vi "Diagnostics.Protocol.Initialize.vi"(8 "error in (no error)":errorcluster, 11 "Parameters":T6={"Properties"={"Name"="", "CAN"={"Interface"="", "Baud Rate"=0, "Diagnostic Protocol"=enum."GMLAN", "Transport Protocol"=enum."ISO TP - Normal Mode", "Transmit ID"=0, "Receive ID"=0, "Transmit Extension"=0, "Receive Extension"=0, "Receive UUDT ID"=0, "Enable Stream"=FALSE, "VW TP Channel ID"=0, "Fill Frame"=FALSE, "Fill Byte"=0, "Termination"=FALSE, "LIN Cluster"="ADCS_LIN_database", "NAD"=1, "IO Mode"=0, "Max DLC"=8, "FD Baud Rate"=0, "Security"={"Type"=enum."None", "Source DLL Path"=path "", "Target DLL Path"=path "", "Security Level"=0, "Master Key"=""}, "Timeout"=0}, "986x"={"Enable"=FALSE, "RIO Device"="", "Bitfile"=path ""}, "Reads"=[], "Frames Lookup"=variant, "Writes"=[], "DPIDs"=[], "DPID Lookup"=variant, "DTC"={"Descriptor"={"DTC Byte Length"=0, "Status Byte Length"=0, "Add Data Byte Length"=0, "Byte Order"=enum."Motorola"}, "Value.Code"=[], "Value.String"=[], "Value.J2012String"=[], "Status.Code"=[], "Status.String"=[]}, "Created DTCs"=0, "Polls"=[], "Service Channels Status Lookup"=variant, "Trigger Lookup"=variant}} {"Properties"."Writes"."Signals"."Byte Order" items=["Little Endian", "Big Endian"]; "Properties"."Writes"."Signals"."Data Type" items=["Signed", "Unsigned", "IEEE Float"]; "Properties"."CAN"."IO Mode" items=["CAN 2.0", "CAN FD", "CAN FD+BRS"]; "Properties"."CAN"."Fill Byte" format="%.0x"; "Properties"."CAN"."VW TP Channel ID" format="%.0x"; "Properties"."CAN"."Receive UUDT ID" format="%.0x"; "Properties"."CAN"."Receive Extension" format="%.0x"; "Properties"."CAN"."Transmit Extension" format="%.0x"; "Properties"."CAN"."Receive ID" format="%.0x"; "Properties"."CAN"."Transmit ID" format="%.0x"; "Properties"."Reads"."Signals"."Byte Order" items=["Little Endian", "Big Endian"]; "Properties"."Reads"."Signals"."Data Type" items=["Signed", "Unsigned", "IEEE Float"]}) -> (0 "error out":errorcluster, 3 "diag ref out":T1={"Diag CAN Handle"=0, "Transport Protocol"=enum."ISO TP - Normal Mode", "Receive Address Extension"=0, "Transmit Address Extension"=0, "Receive CAN Id"=0, "Transmit CAN Id"=0, "Log Frames ?"=FALSE, "My TP Address"=0, "Other TP Address"=0, "T1"=0, "T2"=0, "T3"=0, "T4"=0, "Tx SN"=0, "Block Size"=0, "Rx SN"=0, "VW TP Initialized?"=FALSE, "Tx block no"=0, "baud rate"=0, "Interface"="", "Channel Diag CAN Handle"=0, "UDP Connection ID"=refnum, "TCP Connection ID"=refnum, "Target IP Addr"=0, "Source Address"=0, "Target Address"=0, "Send Header NACK?"=FALSE, "DLL Handle"=0, "NAD"=0, "Time Stamp read first"=0.0, "Time Stamp read last"=0.0, "Time Stamp write first"=0.0, "Time Stamp write last"=0.0, "Time Stamp write"=0.0, "Time Stamp read"=0.0, " I/O Mode"=0, "FD Baudrate"=0, "TX_DL"=8, "RX_DL"=8, "DoIP Protocol Version"=1, " Selected I/O Mode"=0, "TesterPresent Counter"=0, "TesterPresent Limit"=0, "TesterPresent Tick[ms]"=10, "TesterPresent RequireResponse?"=FALSE, "TesterPresent Stored Ref?"=FALSE, "TesterPresent Message"=[], "TesterPresent Task Handle"=0, "TesterPresent Semaphore"=refnum, "Response Plausibility Check"=1, "Default Version?"=TRUE, "Diagostic Globals"={"Timeout FC (Bs)"=250, "Timeout CF (Cr)"=250, "Timeout Diag Command"=1000, "Receive Block Size (BS)"=0, "Wait Time CF (STmin)"=5, "Max Waits (N_WFTmax)"=10, "Waits to Send (N_WAIT)"=0, "Time between Waits (TW)"=25, "Fill CAN Frames?"=TRUE, "Fill Byte"=255, "Invalid Response as Error?"=FALSE, "Max RspPending Count"=5, "VWTP Command Timeout"=50, "Transport Protocol"=enum."Diagnostics on IP", "Diag CAN Handle"=0, "DLL Handle"=0, "Timeout RspPending"=1000}, "Session-based Properties?"=FALSE} {"Diagostic Globals"."Fill Byte" format="%x"; "TesterPresent Message" format="%.0x"; "Selected I/O Mode" items=["CAN", "CAN FD", "CAN FD+BRS", "ECU Determined"]; "DoIP Protocol Version" items=["2010"=1, "2012"=2]; "RX_DL" items=["8"=8, "12"=12, "16"=16, "20"=20, "24"=24, "32"=32, "48"=48, "64"=64]; "TX_DL" items=["8"=8, "12"=12, "16"=16, "20"=20, "24"=24, "32"=32, "48"=48, "64"=64]; "I/O Mode" items=["CAN", "CAN FD", "CAN FD+BRS", "Not yet determined"]})   [LabVIEW 2019, in "Diagnostics Addon Engine.lvlib"]
uses:
  Diagnostics Addon Engine.lvlib
  Shared/Types/SysDef.Compile.ctl
  Shared/Types/SysDef.Compile.Properties.ctl
  Shared/Types/CAN.ctl
  Shared/Types/CAN.Interface.ctl
  Shared/Types/Protocol.ctl
  Shared/Types/Transport.ctl
  Shared/Types/Security.ctl
  Shared/Types/Security.Type.ctl
  Shared/Types/986x.ctl
  Shared/Types/Frame.Compile.ctl
  Shared/Types/Type.ctl
  Shared/Types/Signal.ctl
  Shared/Types/DPID.ctl
  Shared/Types/DPID.Rate.ctl
  Shared/Types/DTC.Settings.ctl
  Shared/Types/DTC.Descriptor.ctl
  Shared/Types/Poll.Compiled.ctl
  <vilib>/Automotive Diagnostic Command Set/Diagnostic Transport.llb/Diag Reference.ctl
  <vilib>/Automotive Diagnostic Command Set/Diagnostic Transport.llb/Transport Protocol Selector.ctl
  <vilib>/Automotive Diagnostic Command Set/Diagnostic Transport.llb/DoIP Protocol Version.ctl
  <vilib>/Automotive Diagnostic Command Set/Diagnostic Transport.llb/Diag Globals.ctl
  <vilib>/Automotive Diagnostic Command Set/Diagnostic Transport.llb/Property ID.ctl
  <vilib>/Automotive Diagnostic Command Set/Diagnostic Transport.llb/VWTP Application Type.ctl
  <vilib>/Automotive Diagnostic Command Set/Diagnostic Transport.llb/DoIP OpenType.ctl
  <vilib>/addons/Automotive Diagnostic Command Set/NI_Automotive Diagnostic Command Set.lvlib
  Shared/Diagnostics Addon Shared.lvlib
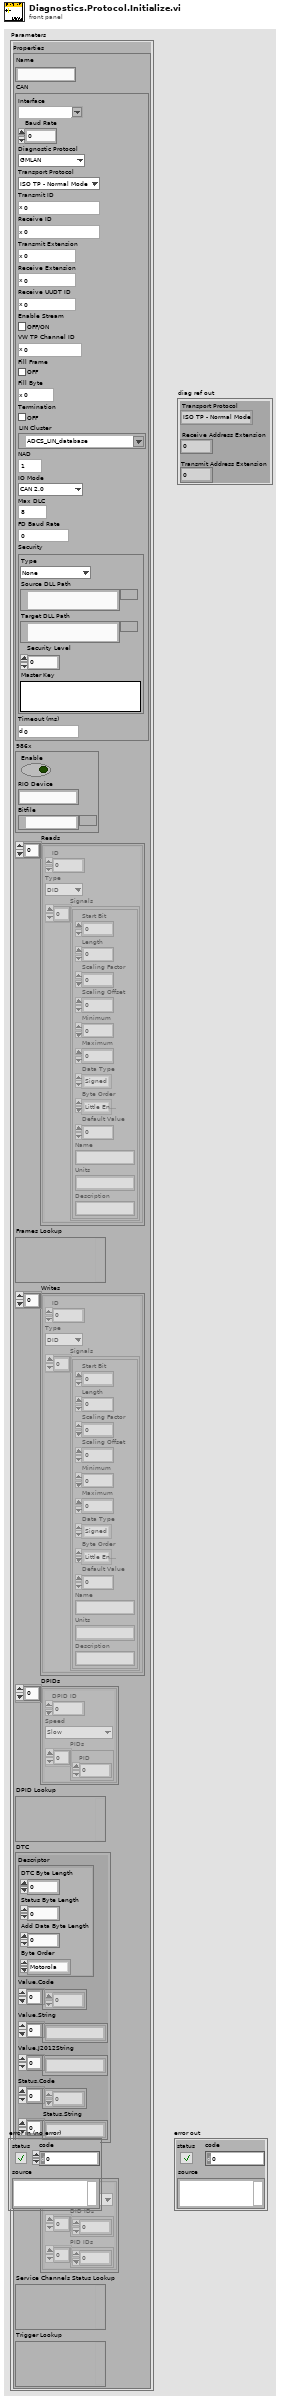
[diagram p1: front panel]
types:
  T1 = typedef "NI_Automotive Diagnostic Command Set.lvlib/Diag Reference.ctl" = cluster{"Diag CAN Handle":u32, "Transport Protocol":T2, "Receive Address Extension":u8, "Transmit Address Extension":u8, "Receive CAN Id":u32, "Transmit CAN Id":u32, "Log Frames ?":bool, "My TP Address":u8, "Other TP Address":u8, "T1":u16, "T2":u16, "T3":u16, "T4":u16, "Tx SN":u8, "Block Size":u8, "Rx SN":u8, "VW TP Initialized?":bool, "Tx block no":u8, "baud rate":u64, "Interface":string, "Channel Diag CAN Handle":u32, "UDP Connection ID":refnum<k16>, "TCP Connection ID":refnum<k5>, "Target IP Addr":u32, "Source Address":u16, "Target Address":u16, "Send Header NACK?":bool, "DLL Handle":u32, "NAD":u8, "Time Stamp read first":dbl, "Time Stamp read last":dbl, "Time Stamp write first":dbl, "Time Stamp write last":dbl, "Time Stamp write":dbl, "Time Stamp read":dbl, " I/O Mode":u32, "FD Baudrate":u64, "TX_DL":u16, "RX_DL":u16, "DoIP Protocol Version":T3, " Selected I/O Mode":u32, "TesterPresent Counter":u32, "TesterPresent Limit":u32, "TesterPresent Tick[ms]":i32, "TesterPresent RequireResponse?":bool, "TesterPresent Stored Ref?":bool, "TesterPresent Message":u8[], "TesterPresent Task Handle":i32, "TesterPresent Semaphore":T4, "Response Plausibility Check":u32, "Default Version?":bool, "Diagostic Globals":T5, "Session-based Properties?":bool}
  T2 = typedef "NI_Automotive Diagnostic Command Set.lvlib/Transport Protocol Selector.ctl" = enum16{"ISO TP - Normal Mode", "ISO TP - Mixed Mode", "VW TP 2.0", "Diagnostics on IP", "ISO TP LIN"}
  T3 = typedef "NI_Automotive Diagnostic Command Set.lvlib/DoIP Protocol Version.ctl" = u8
  T4 = typedef "Semaphore RefNum" = refnum<k1>
  T5 = typedef "NI_Automotive Diagnostic Command Set.lvlib/Diag Globals.ctl" = cluster{"Timeout FC (Bs)":u32, "Timeout CF (Cr)":u32, "Timeout Diag Command":u32, "Receive Block Size (BS)":u8, "Wait Time CF (STmin)":u8, "Max Waits (N_WFTmax)":u8, "Waits to Send (N_WAIT)":i32, "Time between Waits (TW)":u32, "Fill CAN Frames?":bool, "Fill Byte":u32, "Invalid Response as Error?":bool, "Max RspPending Count":u32, "VWTP Command Timeout":u32, "Transport Protocol":T2, "Diag CAN Handle":u32, "DLL Handle":u32, "Timeout RspPending":u32}
  T6 = typedef "Diagnostics Addon Shared.lvlib/SysDef.Compile.ctl" = cluster{"Properties":T7}
  T7 = typedef "Diagnostics Addon Shared.lvlib/SysDef.Compile.Properties.ctl" = cluster{"Name":string, "CAN":T8, "986x":T14, "Reads":T15[], "Frames Lookup":variant, "Writes":T15[], "DPIDs":T18[], "DPID Lookup":variant, "DTC":T20, "Created DTCs":u32, "Polls":T22[], "Service Channels Status Lookup":variant, "Trigger Lookup":variant}
  T8 = typedef "Diagnostics Addon Shared.lvlib/CAN.ctl" = cluster{"Interface":T9, "Baud Rate":u64, "Diagnostic Protocol":T10, "Transport Protocol":T11, "Transmit ID":u32, "Receive ID":u32, "Transmit Extension":u8, "Receive Extension":u8, "Receive UUDT ID":u32, "Enable Stream":bool, "VW TP Channel ID":u32, "Fill Frame":bool, "Fill Byte":u8, "Termination":bool, "LIN Cluster":refnum<k21>, "NAD":u8, "IO Mode":u32, "Max DLC":u16, "FD Baud Rate":u64, "Security":T12, "Timeout":u32}
  T9 = typedef "Diagnostics Addon Shared.lvlib/CAN.Interface.ctl" = string
  T10 = typedef "Diagnostics Addon Shared.lvlib/Protocol.ctl" = enum16{"GMLAN", "KWP-2000", "UDS", "User-Defined"}
  T11 = typedef "Diagnostics Addon Shared.lvlib/Transport.ctl" = enum16{"ISO TP - Normal Mode", "ISO TP - Mixed Mode", "VW TP 2.0", "Diagnostics on IP", "ISO TP LIN"}
  T12 = typedef "Diagnostics Addon Shared.lvlib/Security.ctl" = cluster{"Type":T13, "Source DLL Path":path, "Target DLL Path":path, "Security Level":u8, "Master Key":string}
  T13 = typedef "Diagnostics Addon Shared.lvlib/Security.Type.ctl" = enum16{"None", "DLL", "MasterKey"}
  T14 = typedef "Diagnostics Addon Shared.lvlib/986x.ctl" = cluster{"Enable":bool, "RIO Device":string, "Bitfile":path}
  T15 = typedef "Diagnostics Addon Shared.lvlib/Frame.Compile.ctl" = cluster{"ID":u32, "Type":T16, "Signals":T17[]}
  T16 = typedef "Diagnostics Addon Shared.lvlib/Type.ctl" = enum16{"DID", "CDID", "PID", "CPID", "Read Memory", "Write Memory", "DTC Control", "IO Cmd", "IO Resp", "Routine Start Cmd", "Routine Start Resp", "Routine Request Cmd", "Routine Request Resp", "Routine Stop Cmd", "Routine Stop Resp", "UserDefined Cmd", "UserDefined Rsp", "Tester Present", "Clear DTCs", "Read DTCs", "Start DTCs", "DTC Change Count", "Unlock ECU", "Reset ECU", "Diagnostic Session Control", "Normal Communication Control", "Configure and Start DPIDs", "Stop DPIDs"}
  T17 = typedef "Diagnostics Addon Shared.lvlib/Signal.ctl" = cluster{"Start Bit":u32, "Length":u32, "Scaling Factor":dbl, "Scaling Offset":dbl, "Minimum":dbl, "Maximum":dbl, "Data Type":u32, "Byte Order":u32, "Default Value":dbl, "Name":string, "Units":string, "Description":string}
  T18 = typedef "Diagnostics Addon Shared.lvlib/DPID.ctl" = cluster{"DPID ID":u8, "Speed":T19, "PIDs":u16[]}
  T19 = typedef "Diagnostics Addon Shared.lvlib/DPID.Rate.ctl" = enum16{"Slow", "Medium", "Fast"}
  T20 = typedef "Diagnostics Addon Shared.lvlib/DTC.Settings.ctl" = cluster{"Descriptor":T21, "Value.Code":dbl[], "Value.String":string[], "Value.J2012String":string[], "Status.Code":dbl[], "Status.String":string[]}
  T21 = typedef "Diagnostics Addon Shared.lvlib/DTC.Descriptor.ctl" = cluster{"DTC Byte Length":i32, "Status Byte Length":i32, "Add Data Byte Length":i32, "Byte Order":enum16{"Motorola", "Intel"}}
  T22 = typedef "Diagnostics Addon Shared.lvlib/Poll.Compiled.ctl" = cluster{"Speed":T19, "DID IDs":u32[], "PID IDs":u32[]}
  T23 = typedef "NI_Automotive Diagnostic Command Set.lvlib/Property ID.ctl" = enum16{"Timeout Diag Command", "Timeout FC (Bs)", "Timeout CF (Cr)", "Receive Block Size (BS)", "Wait Time CF (STmin)", "Max Wait Frames (N_WFTmax)", "Wait Frames to Send (N_WAIT)", "Time between Waits (T_W)", "Fill CAN Frames", "Fill Byte", "Invalid Response as Error", "Max RspPending Count", "VWTP Command Timeout", "STmin", "P2min", "Termination", "Timeout RspPending", "LIN Sleep", "Actual CAN IO Mode", "Response Plausibility Check", "Session-based Properties"}
  T24 = typedef "NI_Automotive Diagnostic Command Set.lvlib/VWTP Application Type.ctl" = u8
  T25 = typedef "NI_Automotive Diagnostic Command Set.lvlib/DoIP OpenType.ctl" = u16
  T26 = typedef "NI_Automotive Diagnostic Command Set.lvlib/DoIP Vehicle ID Cluster.ctl" = cluster{"VIN":string, "Source Address":u16, "EID":u8[], "GID":u8[], "IP Address":string, "protocol version":T3}
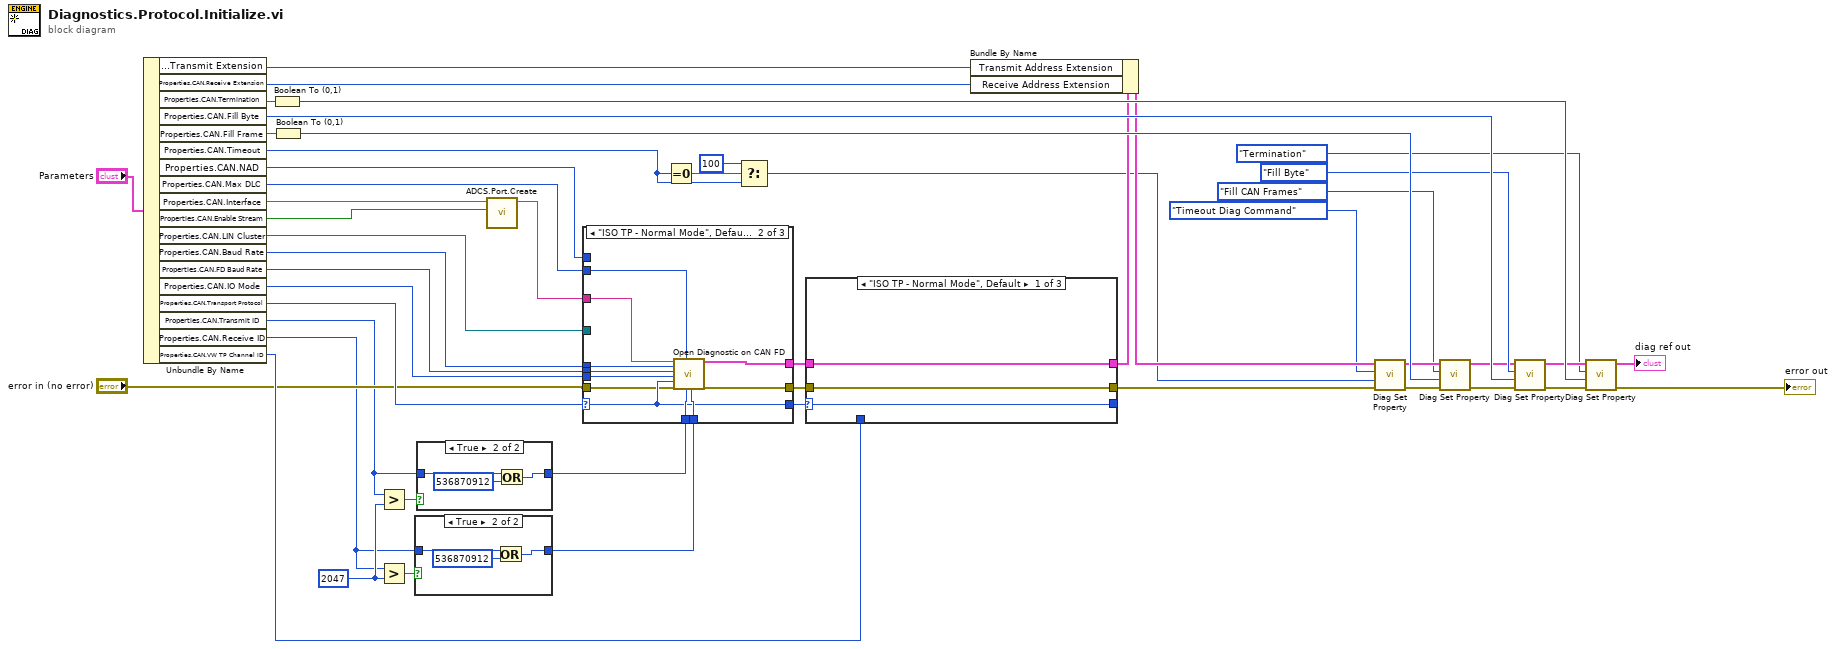
[diagram p0: block diagram]
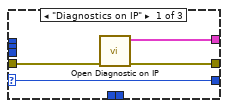
[diagram p4: hidden frame]
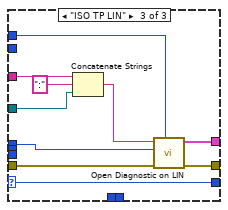
[diagram p5: hidden frame]
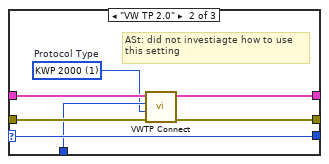
[diagram p6: hidden frame]
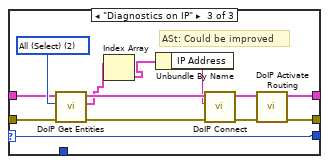
[diagram p7: hidden frame]
diagram:
  w18 = u32 2047 ("y")
  n1 = Unbundle By Name("Parameters") -> ("Properties.CAN.Transmit Extension"=w20:u8, "Properties.CAN.Receive Extension"=w21:u8, "Properties.CAN.Termination"=w45:bool, "Properties.CAN.Fill Byte"=w43:u8, "Properties.CAN.Fill Frame"=w44:bool, "Properties.CAN.Timeout"=w4:u32, "Properties.CAN.NAD"=w11:u8, "Properties.CAN.Max DLC"=w10:u16, "Properties.CAN.Interface"=w19:T9, "Properties.CAN.Enable Stream"=w7:bool, "Properties.CAN.LIN Cluster"=w6:refnum<k21>, "Properties.CAN.Baud Rate"=w49:u64, "Properties.CAN.FD Baud Rate"=w9:u64, "Properties.CAN.IO Mode"=w8:u32, "Properties.CAN.Transport Protocol"=w24:T11, "Properties.CAN.Transmit ID"=w15:u32, "Properties.CAN.Receive ID"=w13:u32, "Properties.CAN.VW TP Channel ID"=w31:u32)
  n2 = Boolean To (0,1)(Boolean=w45) -> (0, 1=w46:i16)
  n3 = Boolean To (0,1)(Boolean=w44) -> (0, 1=w47:i16)
  n4 = Greater?(x=w15, y=w18) -> (0:w17:bool)
  n5 = Greater?(x=w13, y=w18) -> (0:w16:bool)
  n6 = case shown="True" w16 {
    tunnel: w13 -> [w50 w52]
    tunnel: [w50 w51] -> w12
    frame False {
    }
    frame True {
      n7 = Or(x=w52, y=u32 536870912) -> (x .or. y?=w51:u32)
    }
  }
  n8 = case shown="True" w17 {
    tunnel: w15 -> [w54 w57]
    tunnel: [w54 w56] -> w14
    frame False {
    }
    frame True {
      n9 = Or(x=w57, y=u32 536870912) -> (x .or. y?=w56:u32)
    }
  }
  n10 = call "ADCS.Port.Create.vi"("Enable Stream"=w7, "CAN port"=w19) -> ("CAN port out"=w26:string)  [unwired: 9 in]
  n11 = case shown="\"ISO TP - Normal Mode\", Default" w24 {
    selector: w24 -> [w61 w66 w82]
    tunnel: w14 -> [_ w72 _]
    tunnel: w49 -> [_ w71 w80]
    tunnel: w12 -> [_ w70 _]
    tunnel: [w59 w69 w79] -> w27
    tunnel: [w60 w68 w78] -> w29
    tunnel: w26 -> [_ w67 w74]
    tunnel: [w61 w66 w82] -> w25
    tunnel: "error in (no error)" -> [w58 w65 w81]
    tunnel: w11 -> [_ _ w77]
    tunnel: w10 -> [_ w64 _]
    tunnel: w9 -> [_ w63 _]
    tunnel: w8 -> [_ w62 _]
    tunnel: w6 -> [_ _ w75]
    frame "Diagnostics on IP" {
      n12 = call <vilib>:"Open Diagnostic on IP.vi"("error in (no error)"=w58) -> ("error out"=w60:errorcluster, "Diag reference out"=w59:T1)  [unwired: 2 in, 7 out]
    }
    frame "ISO TP - Normal Mode", Default {
      n13 = call <vilib>:"Open Diagnostic on CAN FD.vi"("CAN Interface"=w67, "Baud Rate"=w71, "FD Baud Rate"=w63, "IO Mode"=w62, "Transport Protocol"=w66, "error in (no error)"=w65, "Max DLC"=w64, "Transmit ID"=w72, "Receive ID"=w70) -> ("diag ref out"=w69:T1, "error out"=w68:errorcluster)  [unwired: 9 in]
    }
    frame "ISO TP LIN" {
      n14 = Concatenate Strings(w74, ":" ("string"), w75) -> (w73:string)
      n15 = call <vilib>:"Open Diagnostic on LIN.vi"("NAD"=w77, "error in (no error)"=w81, "Baud Rate"=w80, "Interface"=w73) -> ("error out"=w78:errorcluster, "Diag Ref Out"=w79:T1)  [unwired: 6 in]
    }
  }
  n16 = Equal To 0?(x=w4) -> (x = 0?=w5:bool)
  n17 = Select(t=u32 100, s=w5, f=w4) -> (s? t:f=w2:u32)
  n18 = case shown="\"ISO TP - Normal Mode\", Default" w25 {
    selector: w25 -> [w85 w90 w95]
    tunnel: [w84 w92 w98] -> w28
    tunnel: [w83 w91 w96] -> w30
    tunnel: [w85 w90 w95] -> _
    tunnel: w27 -> [w84 w89 w94]
    tunnel: w29 -> [w83 w88 w93]
    tunnel: w31 -> [_ w87 _]
    frame "ISO TP - Normal Mode", Default {
    }
    frame "VW TP 2.0" {
      w86 = T24 1 items=["KWP 2000"=1, "KS Type 010C"=2, "Infotainment communication"=16, "Application protocol"=32, "WFS/WIV"=33]  # Protocol Type
      # "ASt: did not investiagte how to use\nthis setting"
      n19 = call <vilib>:"VWTP Connect.vi"("error in"=w88, "application type"=w86, "channel ID"=w87, "diag ref in"=w89) -> ("error out"=w91:errorcluster, "diag ref out"=w92:T1)  [unwired: 6 out]
    }
    frame "Diagnostics on IP" {
      w105 = T25 2 items=["VIN", "EID", "All (Select)"] ("DoIP Open Type")
      # "ASt: Could be improved"
      n20 = call <vilib>:"DoIP Get Entities.vi"("error in (no error)"=w93, "DoIP Open Type"=w105, "Diag reference in"=w94) -> ("error out"=w102:errorcluster, "DoIP entities"=w101:T26[], "Diag reference out"=w103:T1)  [unwired: 3 in, 3 out]
      n21 = Index Array(array=w101) -> (element=w100:T26)  [unwired: 1 in]
      n22 = Unbundle By Name(w100) -> ("IP Address"=w99:string)
      n23 = call <vilib>:"DoIP Connect.vi"("error in (no error)"=w102, "address"=w99, "Diag Reference in"=w103) -> ("error out"=w97:errorcluster, "Diag reference out"=w104:T1)  [unwired: 3 in, 4 out]
      n24 = call <vilib>:"DoIP Activate Routing.vi"("error in (no error)"=w97, "Diag reference in"=w104) -> ("error out"=w96:errorcluster, "Diag reference out"=w98:T1)  [unwired: 2 in, 6 out]
    }
  }
  n25 = Bundle By Name(cluster=w28, "Transmit Address Extension"=w20, "Receive Address Extension"=w21) -> (w32:T1)
  n26 = call <vilib>:"Diag Set Property.vi"("error in (no error)"=w30, "property value"=w2, "property ID"=Property_ID."Timeout Diag Command", "diag ref in"=w32) -> ("error out"=w35:errorcluster, "diag ref out"=w40:T1)  [unwired: 6 in]
  n27 = call <vilib>:"Diag Set Property.vi"("error in (no error)"=w35, "property value"=w47, "property ID"=Property_ID."Fill CAN Frames", "diag ref in"=w40) -> ("error out"=w33:errorcluster, "diag ref out"=w1:T1)  [unwired: 6 in]
  n28 = call <vilib>:"Diag Set Property.vi"("error in (no error)"=w33, "property value"=w43, "property ID"=Property_ID."Fill Byte", "diag ref in"=w1) -> ("error out"=w34:errorcluster, "diag ref out"=w41:T1)  [unwired: 6 in]
  n29 = call <vilib>:"Diag Set Property.vi"("error in (no error)"=w34, "property value"=w46, "property ID"=Property_ID."Termination", "diag ref in"=w41) -> ("error out"=→"error out":errorcluster, "diag ref out"=→"diag ref out":T1)  [unwired: 6 in]
